vi "SVG2EMF_Inkscape.vi"(7 "Inkscape.exe":path=path "C:/Program Files (x86)/Inkscape/inkscape.exe", 8 "error in":errorcluster caption="错误输入（无错误）", 10 "emf路径":path, 11 "svg路径":path) -> (0 "error out":errorcluster, 2 "错误？":bool)   [LabVIEW 2018]
doc: "使用inkscape将svg转换成emf"
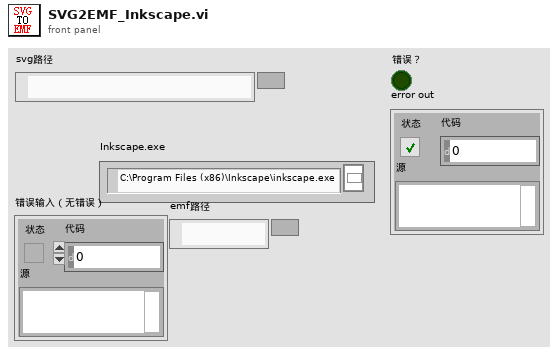
[diagram p1: front panel]
types:
  T1 = enum16{"Null", "NonExist", "EmptyFile", "File", "EmptyDir", "Directory"}
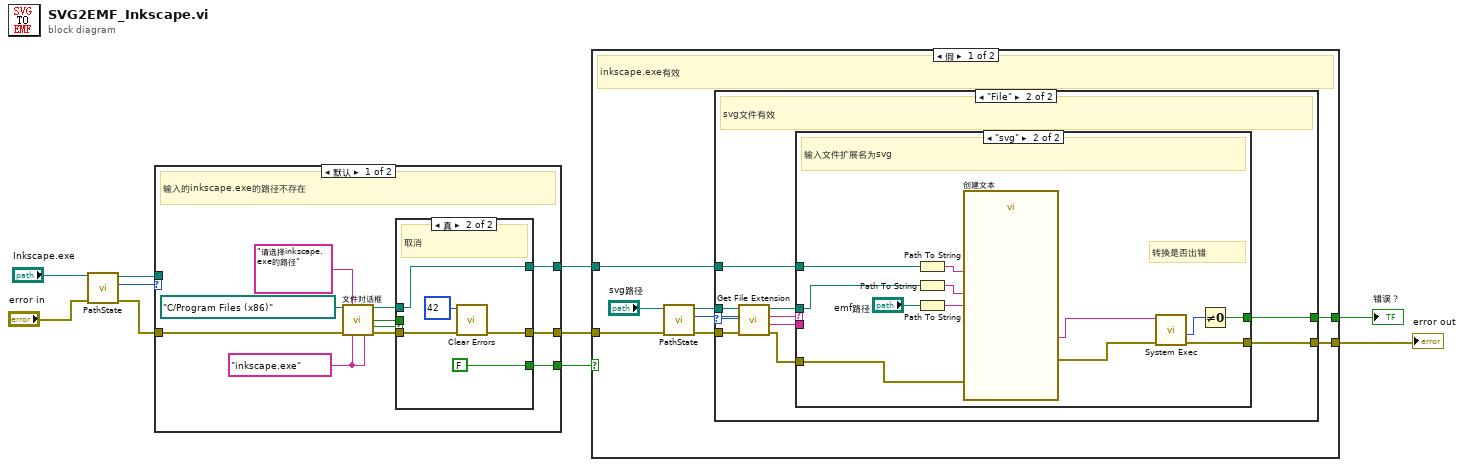
[diagram p0: block diagram]
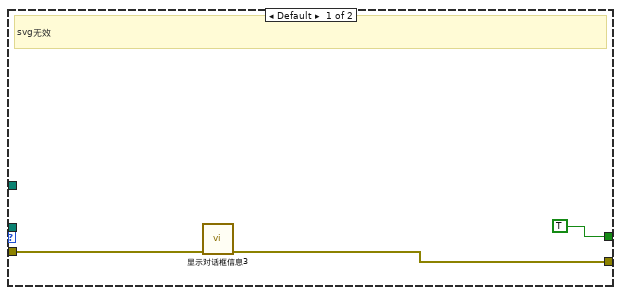
[diagram p2: hidden frame]
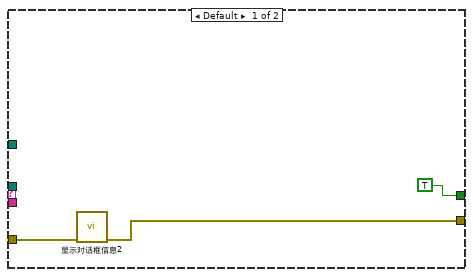
[diagram p3: hidden frame]
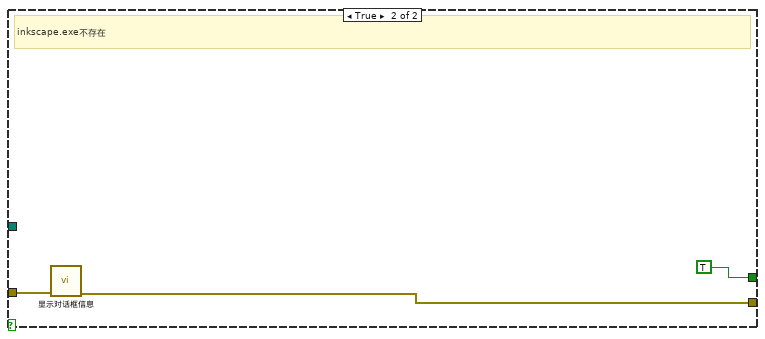
[diagram p4: hidden frame]
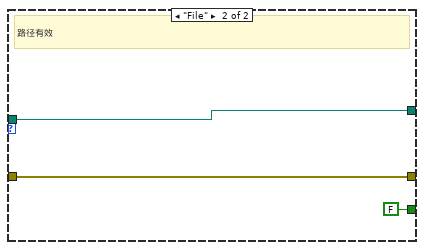
[diagram p6: hidden frame]
diagram:
  n1 = call <vilib>:"PathState.vi"("error in (no error)"="error in", "Path_input"="Inkscape.exe") -> ("error out"=w7:errorcluster, "State"=w9:T1, "Path_output"=w8:path)  [unwired: 7 in]
  n2 = case shown="默认" w9 {
    tunnel: w8 -> [_ w32]
    tunnel: [w12 w32] -> w5
    tunnel: w7 -> [w18 w31]
    tunnel: [w15 w31] -> w4
    tunnel: [w11 FALSE] -> w6
    frame Default {
      w19 = "inkscape.exe" ("default name")
      # "输入的inkscape.exe的路径不存在"
      n3 = call "文件对话框"("start path"=path "C:/Program Files (x86)" ("Inkscape.exe"), "prompt"="请选择inkscape.exe的路径", "error in"=w18, "pattern (all files)"=w19, "pattern label"=w19) -> ("selected path"=w13:path, "exists"=w14:bool, "cancelled"=w17:bool, "error out"=w16:errorcluster)  [unwired: 7 in]
      n4 = case shown="真" w17 {
        tunnel: w16 -> [w24 w29]
        tunnel: [w24 w28] -> w15
        tunnel: w14 -> [w22 _]
        tunnel: w13 -> [w23 w26]
        tunnel: [w23 w26] -> w12
        tunnel: [w22 FALSE] -> w11
        frame False {
          # "选择了有效路径"
        }
        frame True {
          # "取消"
          n5 = call <vilib>:"Clear Errors.vi"("error in (no error)"=w29, "specific error code to clear (0: all)"=42) -> ("error out"=w28:errorcluster)  [unwired: 4 in, 1 out]
        }
      }
    }
    frame "File" {
      # "路径有效"
    }
  }
  n6 = case shown="假" w6 {
    tunnel: w5 -> [w37 _]
    tunnel: w4 -> [w35 w70]
    tunnel: [w34 w69] -> w2
    tunnel: [w33 TRUE] -> w3
    frame False {
      # "inkscape.exe有效"
      n7 = call <vilib>:"PathState.vi"("error in (no error)"=w35, "Path_input"="svg路径") -> ("error out"=w36:errorcluster, "State"=w39:T1, "Path_output"=w38:path)  [unwired: 7 in]
      n8 = case shown="\"File\"" w39 {
        tunnel: w38 -> [_ w50]
        tunnel: w37 -> [_ w52]
        tunnel: w36 -> [w43 w51]
        tunnel: [w42 w45] -> w34
        tunnel: [TRUE w44] -> w33
        frame Default {
          # "svg无效"
          n9 = call "显示对话框信息3"("error in (no error)"=w43) -> ("error out"=w42:errorcluster)  [unwired: 9 in, 1 out]
        }
        frame "File" {
          # "svg文件有效"
          n10 = call <vilib>:"Get File Extension.vi"("error in (no error)"=w51, "file"=w50) -> ("error out"=w46:errorcluster, "filename without extension"=w47:string, "lowercase file extension"=w49:string, "dup file"=w48:path)  [unwired: 5 in, 1 out]
          n11 = case shown="\"svg\"" w49 {
            tunnel: w52 -> [_ w64]
            tunnel: w48 -> [_ w61]
            tunnel: w47 -> [_ _]
            tunnel: w46 -> [w55 w58]
            tunnel: [w53 w66] -> w45
            tunnel: [TRUE w65] -> w44
            frame Default {
              n12 = call "显示对话框信息2"("error in (no error)"=w55) -> ("error out"=w53:errorcluster)  [unwired: 9 in, 1 out]
            }
            frame "svg" {
              # "转换是否出错"
              # "输入文件扩展名为svg"
              n13 = Path To String(path=w64) -> (string=w63:string)
              n14 = Path To String(path=w61) -> (string=w62:string)
              n15 = Path To String(path="emf路径") -> (string=w60:string)
              n16 = call "创建文本"("inkscape"=w63, "SVG"=w62, "EMF"=w60, "error in (no error)"=w58) -> ("Result"=w56:string, "error out"=w57:errorcluster)  [unwired: 10 in]
              n17 = call <vilib>:"System Exec.vi"("error in (no error)"=w57, "command line"=w56) -> ("error out"=w66:errorcluster, "return code"=w67:i32)  [unwired: 6 in, 2 out]
              n18 = Not Equal To 0?(x=w67) -> (x != 0?=w65:bool)
            }
          }
        }
      }
    }
    frame True {
      # "inkscape.exe不存在"
      n19 = call "显示对话框信息"("error in (no error)"=w70) -> ("error out"=w69:errorcluster)  [unwired: 9 in, 1 out]
    }
  }
  "错误？" <- w3
  "error out" <- w2
